vi "Write.vi"(8 "error in (no error)":errorcluster, 10 "Value":T1, 11 "Double Float.lvclass in":refnum<class "DAQmx-Bus_DBL_Type.lvclass">) -> (0 "error out":errorcluster, 3 "Double Float.lvclass out":refnum<class "DAQmx-Bus_DBL_Type.lvclass">)   [LabVIEW 2021, in "DAQmx-Bus_DBL_Type.lvclass"]
doc: "Abstract Data Classes 2.1.1.13\nTim Streeter - TSA\nCopyright (c) 2025, TSA"
uses:
  DAQmx-Bus_DBL_Type.lvclass
  <vilib>/TSA/Abstract Data Classes/Abs_Types/Double Float/Support/Type.ctl
  DAQmx-Bus_DBL_Type.lvclass/DAQmx-Bus_DBL_Type.ctl
  <vilib>/TSA/Abstract Data Classes/Abs_Types/Double Float/Abs_Double Float.lvclass
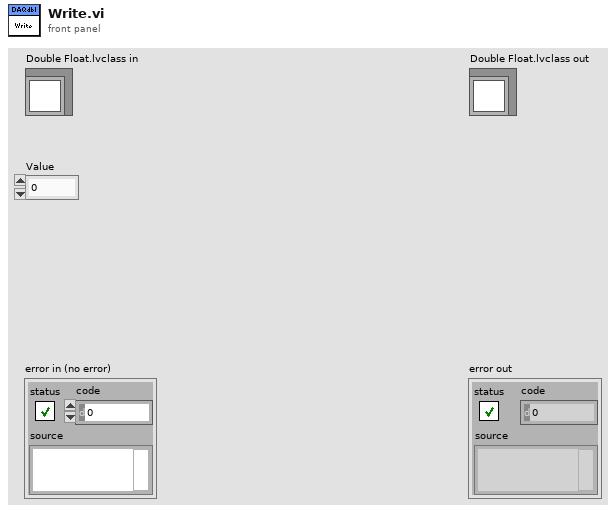
[diagram p1: front panel]
types:
  T1 = typedef "Abs_Double Float.lvclass/Type.ctl" = dbl
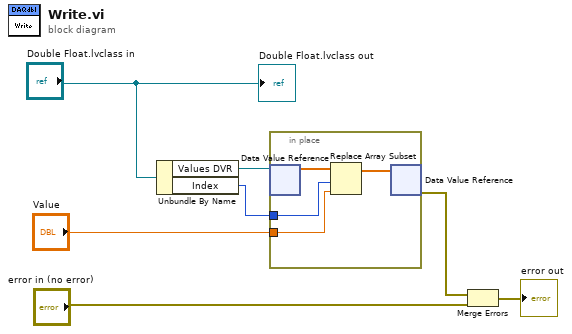
[diagram p0: block diagram]
diagram:
  n1 = Unbundle By Name("Double Float.lvclass in") -> ("Values DVR"=w7:refnum<data-value>, "Index"=w6:i32)
  n2 = in-place {
    in-place-border: w6 -> [w9]
    in-place-border: "Value" -> [w8]
    n3 = in-place-dvr #1(w7) -> (w11:dbl[])  [unwired: 1 out]
    n4 = Replace Array Subset(array=w11, new element=w8, index=w9) -> (w10:dbl[])
    n5 = in-place-dvr #1(w10) -> (w5:errorcluster)  [unwired: 1 out]
  }
  n6 = Merge Errors(w5, "error in (no error)") -> (→"error out":errorcluster)
  "Double Float.lvclass out" <- "Double Float.lvclass in"
